vi "Convert RPC Error to LabVIEW Error.vi"(9 "JSON in":refnum<class "JSON Null.lvclass">, 11 "RPC Error Code":i32) -> (2 "error out":errorcluster)   [LabVIEW 2016, in "JSONRPC Server.lvclass"]
uses:
  JSONRPC Server.lvclass
  <vilib>/NI/JSON Support for LabVIEW/JSON Data Classes/JSON Datatype/JSON Null.lvclass
  <vilib>/NI/JSON Support for LabVIEW/JSON Data Classes/JSON Helper/To More Specific Type (Object).vi
  <vilib>/NI/JSON Support for LabVIEW/JSON Data Classes/JSON Object/Get Value (Numeric Value).vi
  <vilib>/NI/JSON Support for LabVIEW/JSON Data Classes/JSON Object/Get Value (String Value).vi
  <vilib>/NI/JSON Support for LabVIEW/JSON Data Classes/JSON Helper/JSON Helper.lvclass
  <vilib>/NI/JSON Support for LabVIEW/JSON Data Classes/JSON Object/JSON Object.lvclass
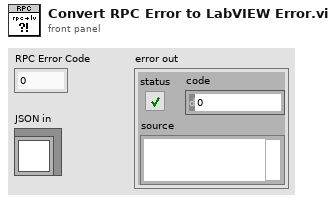
[diagram p1: front panel]
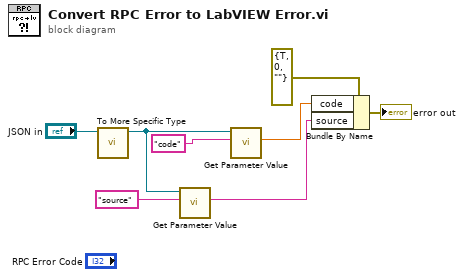
[diagram p0: block diagram]
diagram:
  n1 = call-poly <vilib>:"To More Specific Type.vi"("JSON Datatype in"="JSON in") -> ("JSON Datatype out"=w4:refnum<class "JSON Object.lvclass">)  [unwired: 9 in, 1 out]
  n2 = call-poly <vilib>:"Get Parameter Value.vi"("key"="source", "JSON Object in"=w4) -> ("value"=w1:string)  [unwired: 8 in, 1 out]
  n3 = call-poly <vilib>:"Get Parameter Value.vi"("key"="code" ("Parameter Name"), "JSON Object in"=w4) -> ("value"=w2:dbl)  [unwired: 8 in, 1 out]
  n4 = Bundle By Name(cluster=errorcluster {"status"=TRUE, "code"=0, "source"=""} ("error constant"), "code"=w2, "source"=w1) -> (→"error out":errorcluster)
